vi "Untitled 1.vi"(8 "error in (no error)":errorcluster, 11 "Autofocus in":refnum<class "Autofocus.lvclass">) -> (0 "error out":errorcluster, 3 "Autofocus out":refnum<class "Autofocus.lvclass">)   [LabVIEW 2012, in "Autofocus.lvclass"]
uses:
  Autofocus.lvclass
  Autofocus.lvclass/Autofocus.ctl
  <vilib>/Analysis/NI_AALPro.lvlib
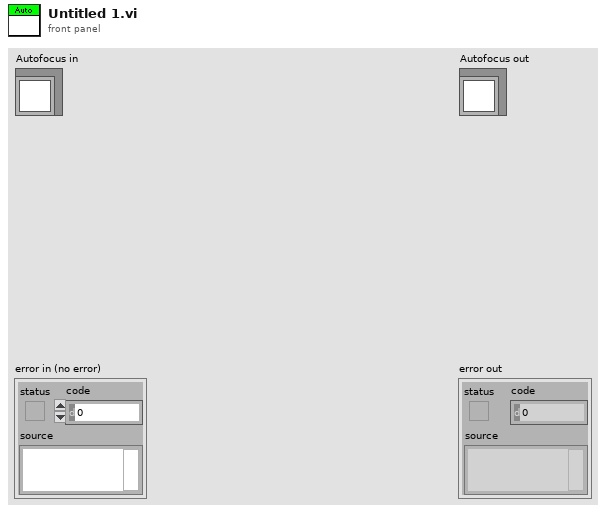
[diagram p1: front panel]
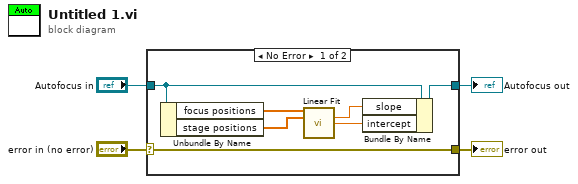
[diagram p0: block diagram]
diagram:
  n1 = case shown="No Error" "error in (no error)" {
    selector: "error in (no error)" -> [w11 w13]
    tunnel: [w11 w13] -> w3
    tunnel: [w7 w12] -> w1
    tunnel: "Autofocus in" -> [w8 w12]
    frame No Error {
      n2 = Unbundle By Name(w8) -> ("focus positions"=w10:dbl[], "stage positions"=w9:dbl[])
      n3 = call <vilib>:"Linear Fit.vi"("Y"=w10, "X"=w9) -> ("slope"=w6:dbl, "intercept"=w5:dbl)  [unwired: 9 in, 3 out]
      n4 = Bundle By Name(cluster=w8, "slope"=w6, "intercept"=w5) -> (w7:refnum<class "Autofocus.lvclass">)
    }
    frame Error {
    }
  }
  "error out" <- w3
  "Autofocus out" <- w1
